vi "HandleRx.vi"(8 "error in (no error)":errorcluster, 11 "Server in":refnum<class "Server.lvclass">) -> (0 "error out":errorcluster, 3 "Server out":refnum<class "Server.lvclass">)   [LabVIEW 2018, in "Server.lvclass"]
uses:
  Server.lvclass
  Server.lvclass/Server.ctl
  Comm/Stream/Stream.lvclass
panel:
  out "MsgRX":string
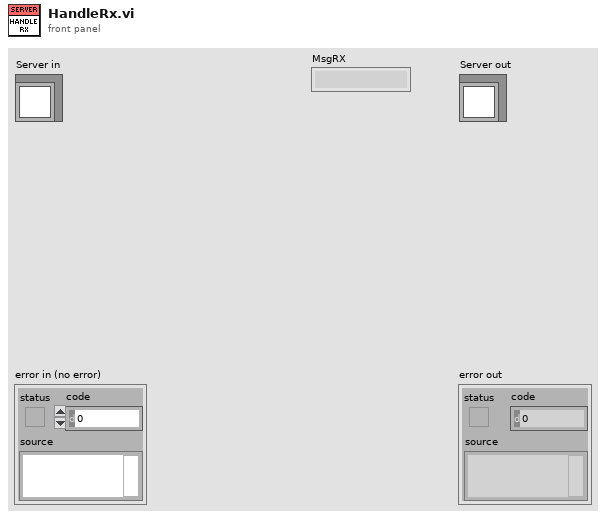
[diagram p1: front panel]
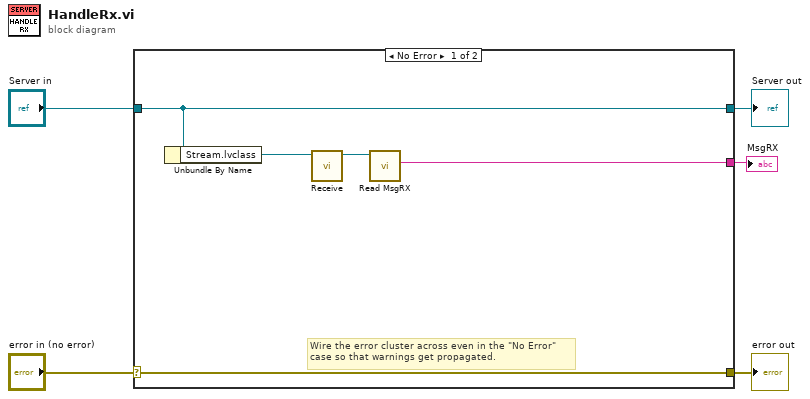
[diagram p0: block diagram]
diagram:
  n1 = case shown="No Error" "error in (no error)" {
    selector: "error in (no error)" -> [w10 w12]
    tunnel: [w10 w12] -> w4
    tunnel: [w8 w11] -> w2
    tunnel: "Server in" -> [w8 w11]
    tunnel: [w6 _] -> w1
    frame No Error {
      # "Wire the error cluster across even in the \"No Error\"\ncase so that warnings get propagated."
      n2 = Unbundle By Name(w8) -> ("Stream.lvclass"=w7:refnum<class "Stream.lvclass">)
      n3 = call-dynamic "Receive.vi"("Stream in"=w7) -> ("Stream out"=w9:refnum<class "Stream.lvclass">)  [unwired: 9 in, 1 out]
      n4 = call-dynamic "Read MsgRX.vi"("Comm in"=w9) -> ("MsgRX"=w6:string)  [unwired: 8 in, 2 out]
    }
    frame Error {
    }
  }
  "error out" <- w4
  "Server out" <- w2
  "MsgRX" <- w1
